vi "SetFileName.vi"(5 "Path":path, 6 "error in":errorcluster, 9 "WebSocket connection":refnum<k5>) -> (0 "error out":errorcluster, 3 "WebSocket connection out":refnum<k5>)   [LabVIEW 2014, in "RasPiDownloader.lvlib"]
uses:
  RasPiDownloader.lvlib
  Websocket/Websocket.lvlib
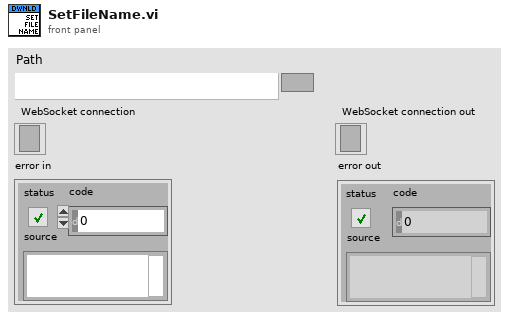
[diagram p1: front panel]
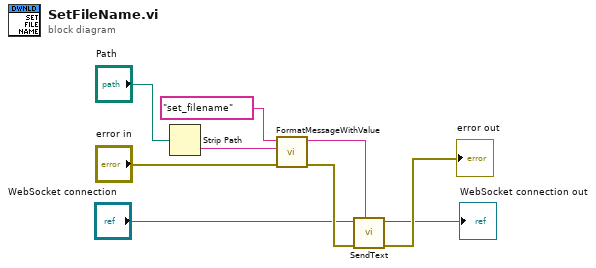
[diagram p0: block diagram]
diagram:
  n1 = Strip Path(path="Path") -> (name=w8:string)  [unwired: 1 out]
  n2 = call "FormatMessageWithValue.vi"("error in"="error in", "value"=w8, "cmd"="set_filename") -> ("error out"=w5:errorcluster, "JSON string"=w6:string)  [unwired: 7 in]
  n3 = call "SendText.vi"("payload"=w6, "error in"=w5, "connection ID"="WebSocket connection") -> ("error out"=→"error out":errorcluster, "connection ID out"=→"WebSocket connection out":refnum<k5>)  [unwired: 5 in]
